vi "IMP_Query.vi"(0 "System no.":i32=1 min=1 max=4 step=1, 2 "Query axis":string, 5 "error in":errorcluster, 6 "Xo":i32, 7 "N":i32=100, 8 "Nmax":i32=1024) -> (14 "Impulse response":dbl[](array[numeric]) format="%.6f", 15 "Impulse size":dbl caption="Numeric" format="%.6f", 19 "error out":errorcluster)   [LabVIEW 2020]
doc: "GCS 1.0 controller: Returns N saved impulse response points. N must be less than or equal to Nmax. For large N values, communication timeout must be set long enough, otherwise a comm.error may occur.\nGCS 2.0 or higher: Returns IMP settings. Use DRR? to read impulse response points back.\n\nE-517, E-518, E-709, E-754, E-755: xo, N and Nmax are not valid. VI reads impulse size. Impulse response is not valid.\n\nE-710: Nmax = 32256. VI reads impulse response points. Impulse size is not valid. \n\nE-761: Nmax = 8192. VI reads impulse response points. Impulse size is not valid."
uses:
  Global1.vi
panel:
  # "GCS 1.0 controller: Returns N saved impulse response points. N must be \nless than or equal to Nmax. For large N values, communication timeout \nmust be set long enough, otherwise a comm.error may occur.\nGCS 2.0 or higher: Returns IMP settings. Use DRR? to read impulse response \npoints back."
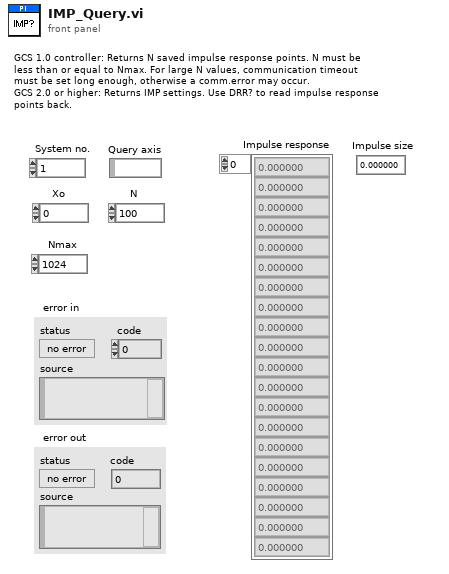
[diagram p1: front panel]
types:
  T1 = typedef "Syntax.ctl" = enum16{"GCS 1.0", "GCS 2.0", "GCS 3.0"}
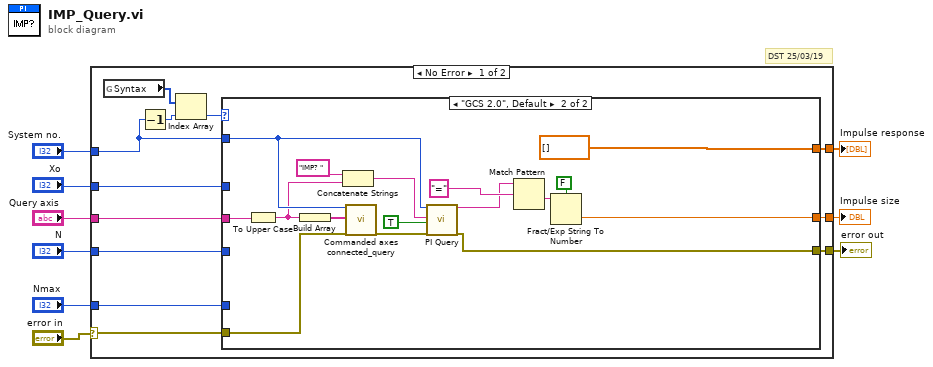
[diagram p0: block diagram]
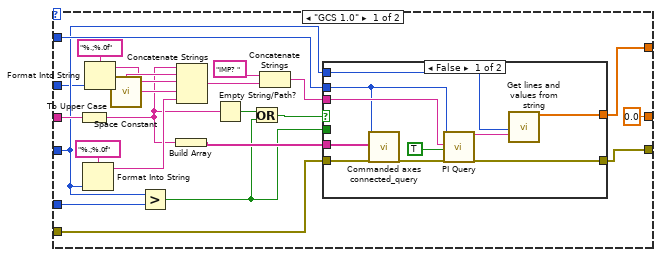
[diagram p2: hidden frame]
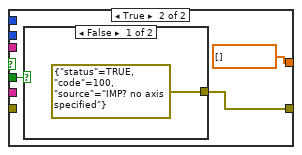
[diagram p3: hidden frame]
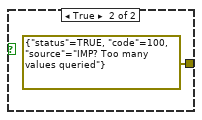
[diagram p4: hidden frame]
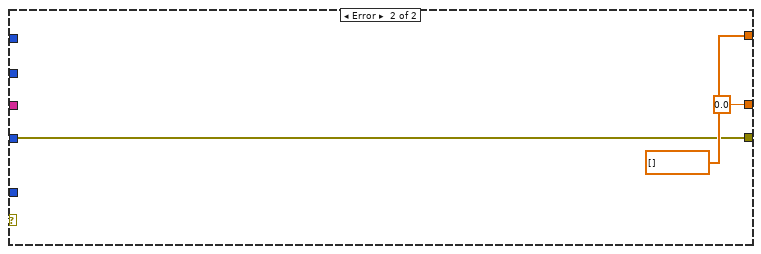
[diagram p5: hidden frame]
diagram:
  # "DST 25/03/19"
  n1 = case shown="No Error" "error in" {
    selector: "error in" -> [w14 w75]
    tunnel: "System no." -> [w11 _]
    tunnel: "Query axis" -> [w21 _]
    tunnel: [w20 w75] -> w8
    tunnel: [w19 dbl[] []] -> w7
    tunnel: "N" -> [w18 _]
    tunnel: "Xo" -> [w17 _]
    tunnel: "Nmax" -> [w16 _]
    tunnel: [w15 0.0] -> w2
    frame No Error {
      n2 = global read "Global1.vi" "Syntax"() -> (w13:T1[])
      n3 = Decrement(x=w11) -> (x-1=w12:i32)
      n4 = Index Array(array=w13, index=w12) -> (element=w10:T1)
      n5 = case shown="\"GCS 2.0\", Default" w10 {
        tunnel: w11 -> [w41 w71]
        tunnel: w21 -> [w39 w73]
        tunnel: [w37 w59] -> w20
        tunnel: [w36 dbl[] []] -> w19
        tunnel: w18 -> [w35 _]
        tunnel: w17 -> [w33 _]
        tunnel: w16 -> [w29 _]
        tunnel: w14 -> [w24 w67]
        tunnel: [0.0 w62] -> w15
        frame "GCS 1.0" {
          n6 = To Upper Case(1:w39) -> (0:w22:string)
          n7 = Format Into String(format string="%.;%.0f" ("Format String"), w35) -> (resulting string=w30:string)  [unwired: 2 in, 1 out]
          n8 = Format Into String(format string="%.;%.0f" ("Format String"), w33) -> (resulting string=w31:string)  [unwired: 2 in, 1 out]
          n9 = call "Space Constant.vi"() -> ("String"=w32:string)
          n10 = Greater?(x=w35, y=w29) -> (0:w25:bool)
          n11 = Build Array(w22) -> (w40:string[])
          n12 = Concatenate Strings(w22, w32, w31, w32, w30) -> (w23:string)
          n13 = Empty String/Path?(string/path=w22) -> (empty?=w27:bool)
          n14 = Or(x=w27, y=w25) -> (x .or. y?=w26:bool)
          n15 = Concatenate Strings("IMP? ", w23) -> (w42:string)
          n16 = case shown="False" w26 {
            tunnel: w42 -> [w52 _]
            tunnel: w41 -> [w51 _]
            tunnel: w40 -> [w50 _]
            tunnel: [w44 w54] -> w37
            tunnel: w35 -> [w48 _]
            tunnel: [w49 dbl[] [] ("Waveform points")] -> w36
            tunnel: w25 -> [_ w55]
            tunnel: w24 -> [w46 _]
            frame False {
              n17 = call "Commanded axes connected_query.vi"("System no."=w51, "Commanded axes"=w50, "error in"=w46) -> ("error out"=w47:errorcluster)  [unwired: 1 in, 15 out]
              n18 = call "PI Query.vi"("System no."=w51, "String to send"=w52, "Attach termination char.?"=TRUE ("Attach Linefeed?"), "error in"=w47) -> ("String read"=w45:string, "error out"=w44:errorcluster)  [unwired: 3 in, 11 out]
              n19 = call "Get lines and values from string.vi"("Array size"=w48, "Input string"=w45) -> ("Numerical values"=w49:dbl[])  [unwired: 17 out]
            }
            frame True {
              n20 = case shown="False" w55 {
                tunnel: [errorcluster {"status"=TRUE, "code"=100, "source"="IMP? no axis specified"} ("error out") errorcluster {"status"=TRUE, "code"=100, "source"="IMP? Too many values queried"} ("error out")] -> w54
                frame False {
                }
                frame True {
                }
              }
            }
          }
        }
        frame "GCS 2.0", Default {
          n21 = To Upper Case(1:w73) -> (0:w66:string)
          n22 = Build Array(w66) -> (w72:string[])
          n23 = Concatenate Strings("IMP? ", w66) -> (w69:string)
          n24 = call "Commanded axes connected_query.vi"("System no."=w71, "Commanded axes"=w72, "error in"=w67) -> ("error out"=w68:errorcluster)  [unwired: 1 in, 15 out]
          n25 = call "PI Query.vi"("System no."=w71, "String to send"=w69, "Attach termination char.?"=TRUE ("Attach Linefeed?"), "error in"=w68) -> ("String read"=w60:string, "error out"=w59:errorcluster)  [unwired: 3 in, 11 out]
          n26 = Match Pattern(string=w60, regular expression="=") -> (after substring=w61:string)  [unwired: 4 out]
          n27 = Fract/Exp String To Number(use system decimal point (T)=FALSE, string=w61) -> (number=w62:dbl)  [unwired: 3 out]
        }
      }
    }
    frame Error {
    }
  }
  "error out" <- w8
  "Impulse response" <- w7
  "Impulse size" <- w2
